vi "getSamplingFsMode.vi"(8 "error in (no error)":errorcluster, 11 "Instrument.LockinAPI in":refnum<class "Instrument.LockinAPI.lvclass">) -> (0 "error out":errorcluster, 2 "Fs Mode":T1, 3 "Instrument.LockinAPI out":refnum<class "Instrument.LockinAPI.lvclass">)   [LabVIEW 2019, in "Instrument.LockinAPI.lvclass"]
doc: "API to get the configured sampling mode\n\nIf address=\"\", this API reads from localhost\nIf address is remote lockin, you need to add this computer to allowed whitelist on the lockin computer you are trying to access."
uses:
  Instrument.LockinAPI.lvclass
  Typedefs/LockinAPI.Sampling.FsMode--enum.ctl
  Typedefs/LockinAPI.Commands--Enum.ctl
  893f89ae-de74-4b3b-b6c4-5084387309ab.vi
  893f89ae-de74-4b3b-b6c4-5084387309ab.vi/dc321488-4959-4ea3-8967-933bf2fe6e0d.vi
  893f89ae-de74-4b3b-b6c4-5084387309ab.vi/b9490a8f-748f-402b-af06-f0eac09c0cfc.vi
  <vilib>/Utility/Data Type/Get Type Information.vi
  <vilib>/JDP Science/JSONtext/JSON text to Variant.vi
  <vilib>/JDP Science/JSONtext/LVClass Serializer/JSONtext LVClass Serializer.lvclass
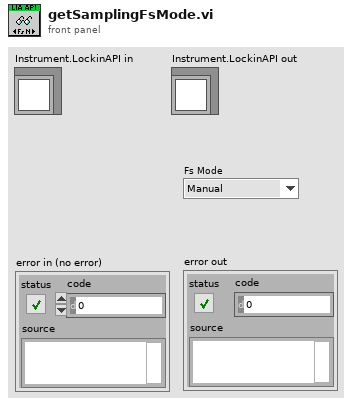
[diagram p1: front panel]
types:
  T1 = typedef "Instrument.LockinAPI.lvclass/LockinAPI.Sampling.FsMode--enum.ctl" = enum16{"Manual", "Auto Fs", "Max Fs"}
  T2 = typedef "Instrument.LockinAPI.lvclass/LockinAPI.Commands--Enum.ctl" = enum16{"setAI", "setAO", "setAO_Amplitude", "setAO_DC", "setAO_Frequency", "setAO_Phase", "setAO_Function", "setREF", "setREF_Frequency", "setREF_Phase", "setREF_TC", "setREF_Roll-Off", "setDAQ", "setSampling", "setOffset", "setState", "getState", "getAO", "getAI", "getResults", "getSampling", "getAOconfig", "getREFconfig", "setInputGain", "setOutputGain", "getInputGain", "getOutputGain", "setSamplingFsMode", "getSamplingFsMode", "setSweep", "setSweep_Time", "setSweep_Table", "getStatus", "getSweepResults", "getSweepWaveforms", "startSweep", "stopSweep"}
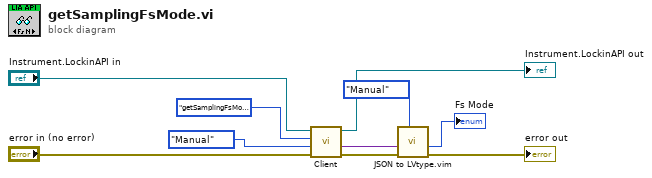
[diagram p0: block diagram]
diagram:
  n1 = call-dynamic "Client.vi"("error in (no error)"="error in (no error)", "Data in"=LockinAPI.Sampling.FsMode--enum."Manual" ("Fs Mode"), "Command in"=LockinAPI.Commands--Enum."getSamplingFsMode" ("Command"), "Instrument in"="Instrument.LockinAPI in") -> ("error out"=w3:errorcluster, "Data out"=w4:variant, "Instrument out"=→"Instrument.LockinAPI out":refnum<class "Instrument.LockinAPI.lvclass">)  [unwired: 4 in, 1 out]
  n2 = call "JSON to LVtype.vim"("type"=LockinAPI.Sampling.FsMode--enum."Manual" ("FsMode"), "error in (no error)"=w3, "JSON Data in"=w4) -> ("error out"=→"error out":errorcluster, "Data out"=→"Fs Mode":T1)  [unwired: 7 in]
